vi "EXIT.vi"() -> ()   [LabVIEW 2019]
panel:
  out "EXIT":bool
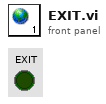
[diagram p1: front panel]
diagram:
